vi "Set Oscillator Sweep Rate.vi"(8 "error in (no error)":errorcluster, 10 "Oscillator Sweep Rate (seconds/step)":dbl min=0.0 max=250000.0 step=0.001, 11 "VISA resource name":refnum<visa-resource-name>) -> (0 "error out":errorcluster, 3 "VISA resource name out":refnum<visa-resource-name>)   [LabVIEW 2016, in "SR7270 Drivers.lvlib"]
uses:
  SR7270 Drivers.lvlib
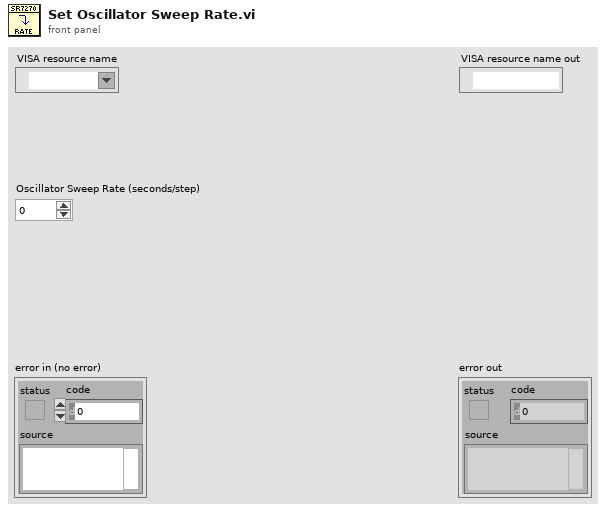
[diagram p1: front panel]
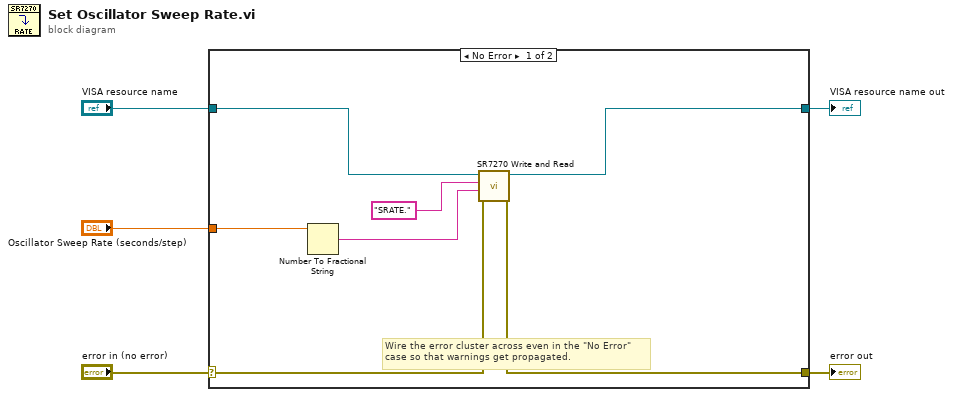
[diagram p0: block diagram]
diagram:
  n1 = case shown="No Error" "error in (no error)" {
    selector: "error in (no error)" -> [w12 w14]
    tunnel: [w11 w14] -> w4
    tunnel: [w6 w13] -> w2
    tunnel: "VISA resource name" -> [w7 w13]
    tunnel: "Oscillator Sweep Rate (seconds/step)" -> [w10 _]
    frame No Error {
      # "Wire the error cluster across even in the \"No Error\"\ncase so that warnings get propagated."
      n2 = Number To Fractional String(number=w10) -> (F-format string=w8:string)  [unwired: 3 in]
      n3 = call "SR7270 Write and Read.vi"("error in (no error)"=w12, "Parameter(s)"=w8, "Command Name"="SRATE.", "VISA resource name"=w7) -> ("error out"=w11:errorcluster, "VISA resource name out"=w6:refnum<visa-resource-name>)  [unwired: 4 in, 2 out]
    }
    frame Error {
    }
  }
  "error out" <- w4
  "VISA resource name out" <- w2
